vi "save_csv_file.vi"(7 "Data":dbl[][](array[numeric]), 8 "error in":errorcluster, 9 "select_out_graph":T1, 10 "Graph":string, 11 "Path":path) -> (0 "error out":errorcluster)   [LabVIEW 2020]
uses:
  ctrl/select_out.ctl
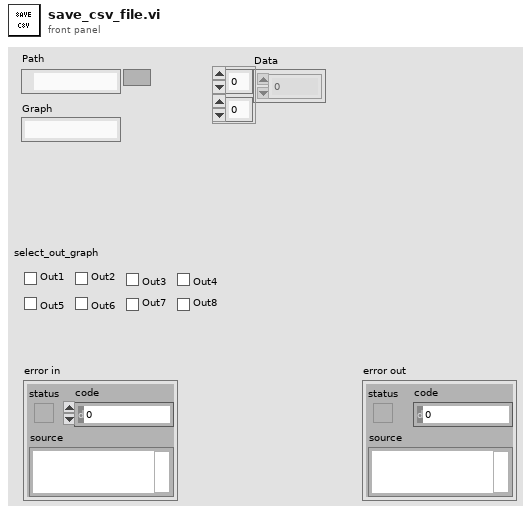
[diagram p1: front panel]
types:
  T1 = typedef "select_out.ctl" = cluster{"out1":bool, "out2":bool, "out3":bool, "out4":bool, "out5":bool, "out6":bool, "out7":bool, "out8":bool}
  T2 = enum16{"open", "replace", "create", "open or create", "replace or create", "replace or create with confirmation"}
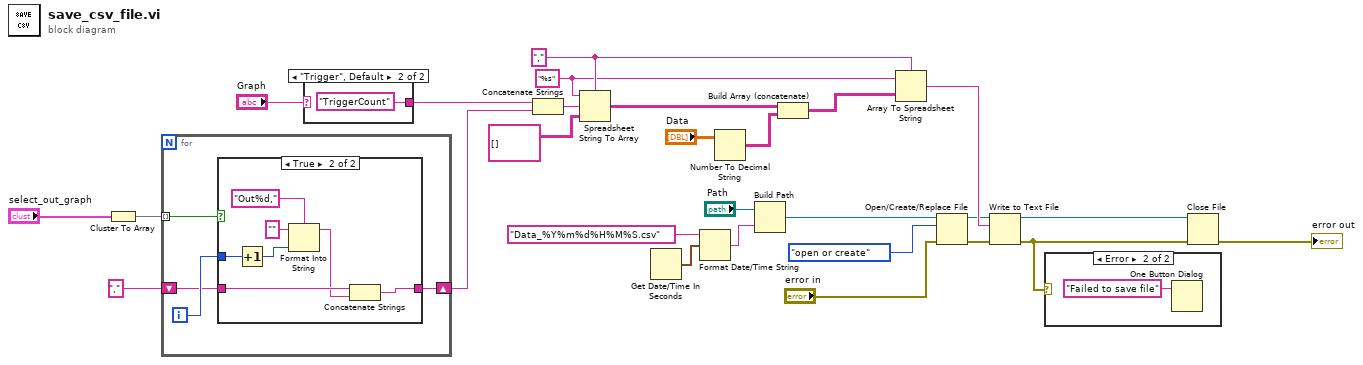
[diagram p0: block diagram]
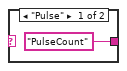
[diagram p3: hidden frame]
diagram:
  w19 = ","
  w16 = "%s"
  n1 = Cluster To Array(cluster="select_out_graph") -> (array=w25:bool[])
  n2 = for {
    tunnel: w25 -> [w31] mode=indexing
    shift-right: [w28] -> w27
    shift-left: "," -> [w29]
    i -> [w30]
    n3 = case shown="True" w31 {
      tunnel: w30 -> [_ w39]
      tunnel: w29 -> [w32 w35]
      tunnel: [w32 w33] -> w28
      frame False {
      }
      frame True {
        n4 = Increment(x=w39) -> (x+1=w38:i32)
        n5 = Format Into String(format string="Out%d,", initial string="", w38) -> (resulting string=w34:string)  [unwired: 1 in, 1 out]
        n6 = Concatenate Strings(w35, w34) -> (w33:string)
      }
    }
  }
  n7 = case shown="\"Trigger\", Default" "Graph" {
    tunnel: ["PulseCount" "TriggerCount"] -> w18
    frame "Pulse" {
    }
    frame "Trigger", Default {
    }
  }
  n8 = Concatenate Strings(w18, w27) -> (w17:string)
  n9 = Spreadsheet String To Array(delimiter (Tab)=w19, format string=w16, spreadsheet string=w17, array type (2D Dbl)=string[][] []) -> (array=w20:string[][])
  n10 = Get Date/Time In Seconds() -> (seconds since 1Jan1904=w2:timestamp)
  n11 = Format Date/Time String(time format string (%c)="Data_%Y%m%d%H%M%S.csv", seconds (now)=w2) -> (date/time string=w12:string)  [unwired: 1 in]
  n12 = Number To Decimal String(number="Data") -> (decimal integer string=w22:string[][])  [unwired: 1 in]
  n13 = Build Path(base path="Path", name or relative path=w12) -> (appended path=w4:path)
  n14 = Build Array (concatenate)(w20, w22) -> (w21:string[][])
  n15 = Array To Spreadsheet String(delimiter (Tab)=w19, array=w21, 3:w16) -> (spreadsheet string=w15:string)
  n16 = Open/Create/Replace File(file path (use dialog)=w4, error in="error in", operation (0:open)=T2."open or create") -> (refnum out=w9:refnum<file>, error out=w6:errorcluster)  [unwired: 3 in, 1 out]
  n17 = Write to Text File(file (use dialog)=w9, text=w15, error in=w6) -> (refnum out=w10:refnum<file>, error out=w11:errorcluster)  [unwired: 1 in, 1 out]
  n18 = case shown="Error" w11 {
    frame No Error {
    }
    frame Error {
      n19 = One Button Dialog(message="Failed to save file") -> ()  [unwired: 1 in, 1 out]
    }
  }
  n20 = Close File(refnum=w10, error in=w11) -> (error out=→"error out":errorcluster)  [unwired: 1 out]
